vi "Measurement Main.vi"() -> ()   [LabVIEW 2017]
uses:
  Controls/saveDataOption.ctl
  TypeDefs/Trav-Command-TD.ctl
  Globals/measurementGlobal.vi
  <vilib>/Utility/file.llb/Read Delimited Spreadsheet (I64).vi
panel:
  in  "Boolean":bool
  in  "Trav Command":T1 items=["Set Reference", "Read Position", "Move", "StopMotors"]
  out "Traverse Position":i32[][](array[numeric])
  out "Block Index":i32
  in  "Setup":enum16{"Run Programme", "Show Setup"}(ring)
  in  "Data Acquisition":T2(ring)
  in  "Save Data Option":T3
  in  "Tap Control":enum32{"Plots", "Status and File"}(tab)
  out "Raw Signals":dbl[][](graph)
  in  "Folder Path":path
  out "Comments":string
  # "ON"
  # "OFF"
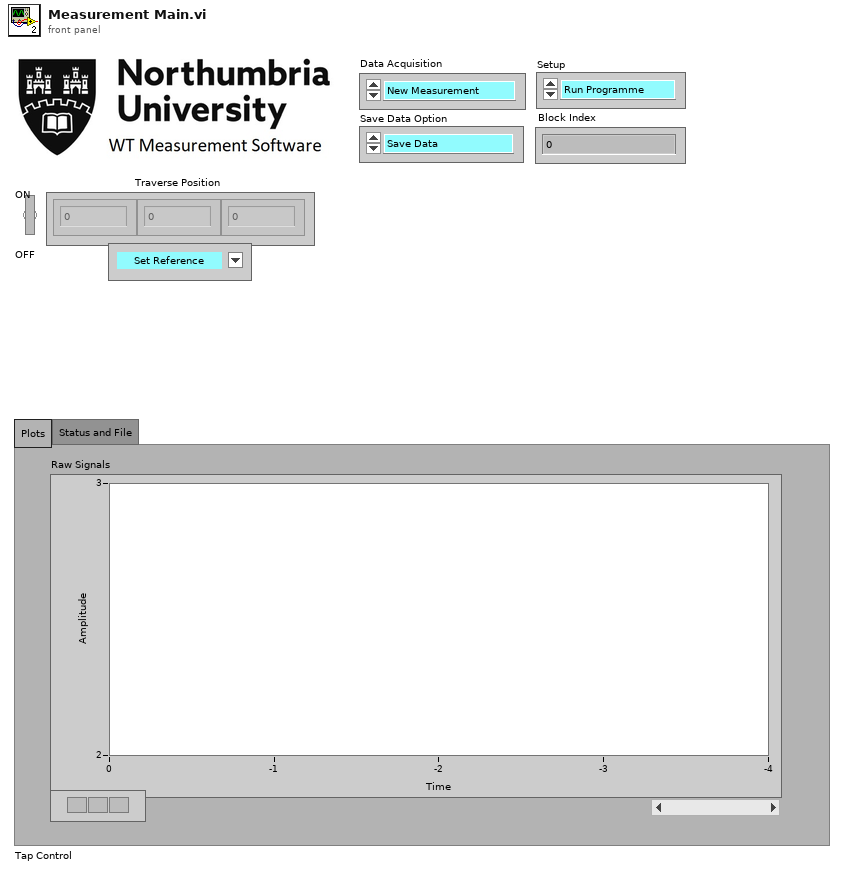
[diagram p1: front panel]
types:
  T1 = typedef "Trav-Command-TD.ctl" = u16
  T2 = enum16{"New Measurement", "Post-process Raw Data"}
  T3 = typedef "saveDataOption.ctl" = enum16{"Save Data", "Do Not Save Data"}
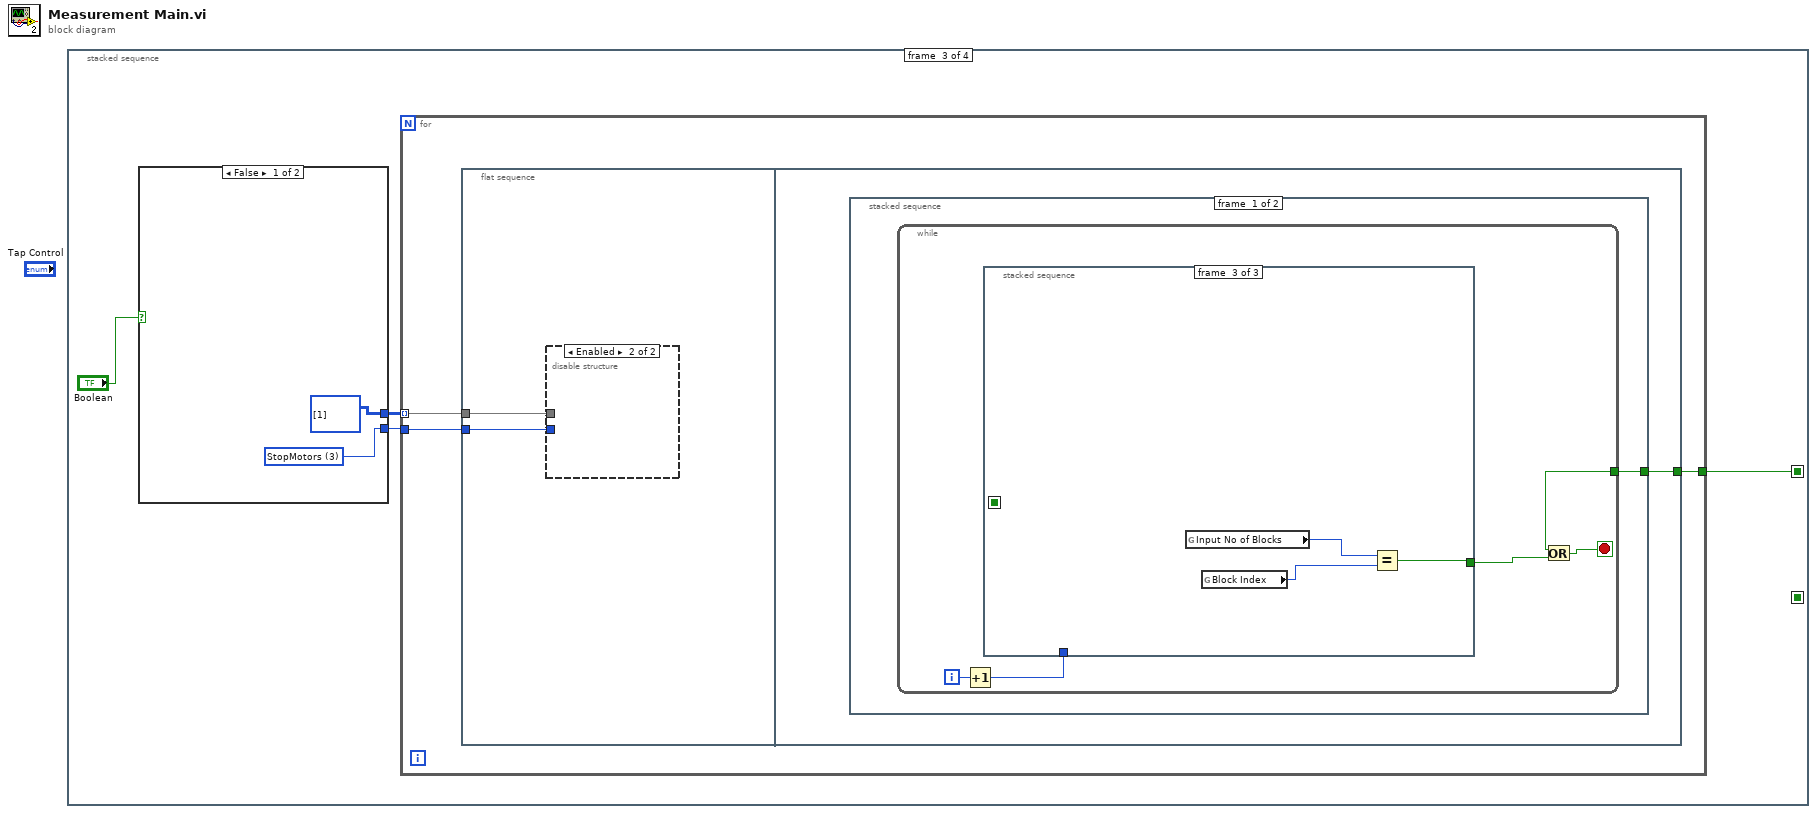
[diagram p0: block diagram]
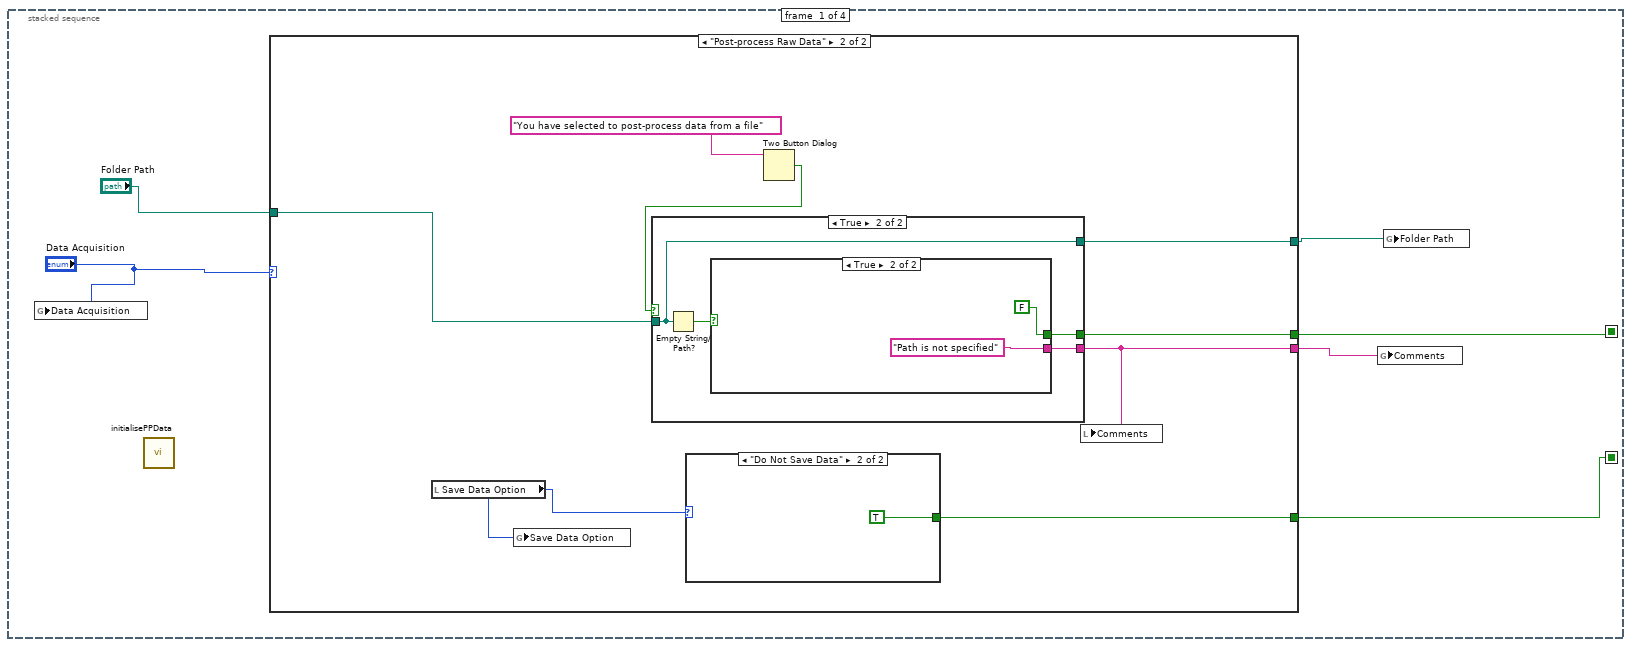
[diagram p2: hidden frame]
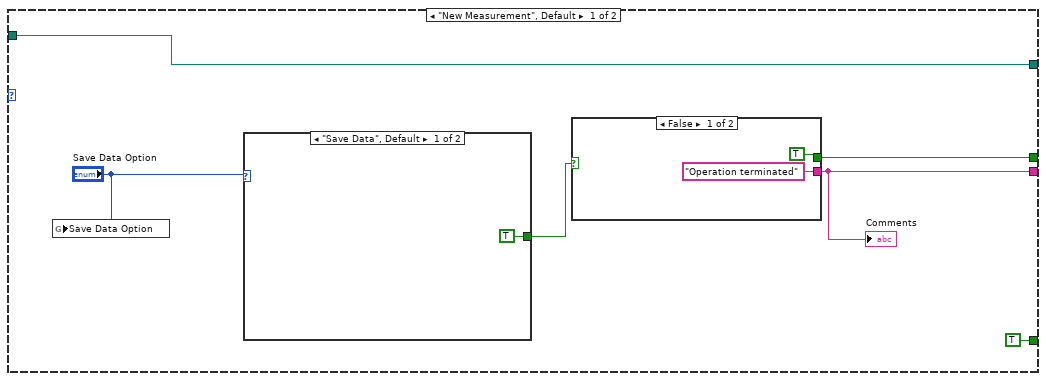
[diagram p3: hidden frame]
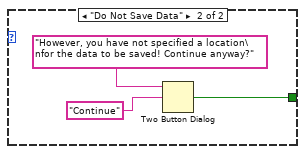
[diagram p4: hidden frame]
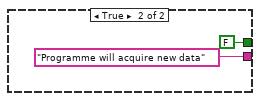
[diagram p5: hidden frame]
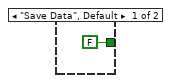
[diagram p6: hidden frame]
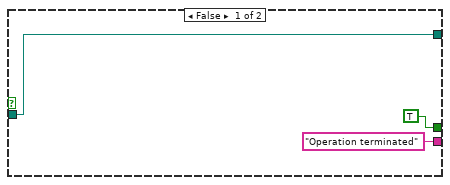
[diagram p7: hidden frame]
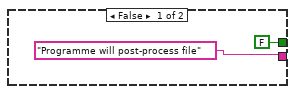
[diagram p8: hidden frame]
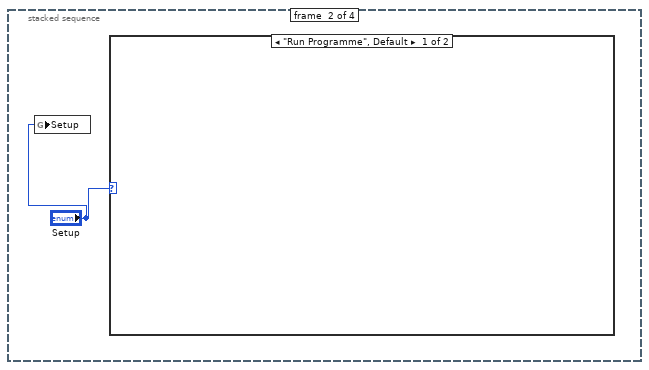
[diagram p9: hidden frame]
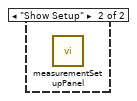
[diagram p10: hidden frame]
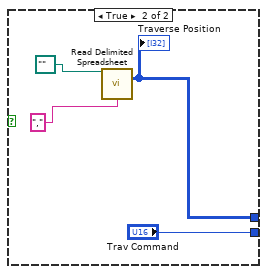
[diagram p11: hidden frame]
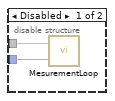
[diagram p12: hidden frame]
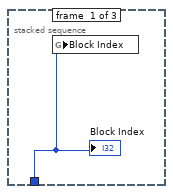
[diagram p13: hidden frame]
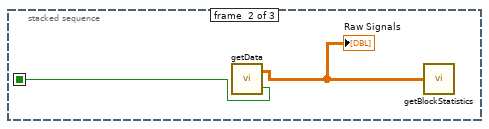
[diagram p14: hidden frame]
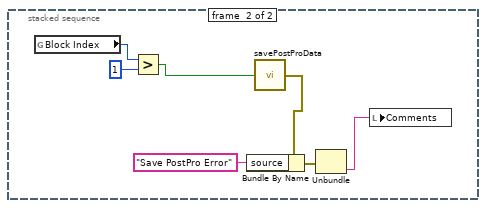
[diagram p15: hidden frame]
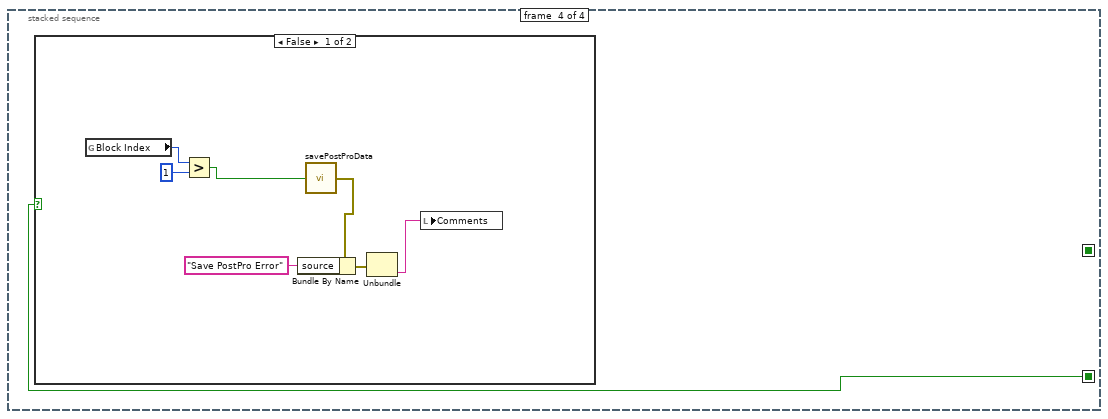
[diagram p16: hidden frame]
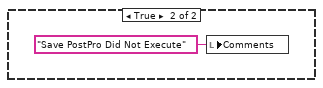
[diagram p17: hidden frame]
diagram:
  n1 = stacked-sequence {
    seq-local: [w4 _ _ _] -> [_ _ w46 _]
    seq-local: [w1 _ _ _] -> [_ _ _ w80]
    frame #0 {
      n2 = global write "measurementGlobal.vi" "Data Acquisition"("Data Acquisition") -> ()
      n3 = call "initialisePPData.vi"() -> ()  [unwired: 12 in]
      n4 = case shown="\"Post-process Raw Data\"" "Data Acquisition" {
        tunnel: [w10 w23] -> w6
        tunnel: [w12 w24] -> w4
        tunnel: "Folder Path" -> [w11 w26]
        tunnel: [w11 w25] -> w5
        tunnel: [TRUE w21] -> w1
        frame "New Measurement", Default {
          n5 = global write "measurementGlobal.vi" "Save Data Option"("Save Data Option") -> ()
          n6 = case shown="\"Save Data\", Default" "Save Data Option" {
            tunnel: [TRUE ("T button?") w15] -> w8
            frame "Save Data", Default {
            }
            frame "Do Not Save Data" {
              n7 = Two Button Dialog(message="However, you have not specified a location\nfor the data to be saved! Continue anyway?", 2:"Continue" ("T button name (\"OK\")")) -> (T button?=w15:bool)  [unwired: 1 in]
            }
          }
          n8 = case shown="False" w8 {
            tunnel: ["Operation terminated" ("Comments") "Programme will acquire new data" ("Comments")] -> w10
            tunnel: [TRUE FALSE] -> w12
            frame False {
            }
            frame True {
            }
          }
          "Comments" <- w10
        }
        frame "Post-process Raw Data" {
          n9 = local read "Save Data Option"() -> (w22:T3)
          n10 = global write "measurementGlobal.vi" "Save Data Option"(w22) -> ()
          n11 = case shown="\"Do Not Save Data\"" w22 {
            tunnel: [FALSE TRUE] -> w21
            frame "Save Data", Default {
            }
            frame "Do Not Save Data" {
            }
          }
          n12 = Two Button Dialog(message="You have selected to post-process data from a file") -> (T button?=w27:bool)  [unwired: 2 in]
          n13 = case shown="True" w27 {
            tunnel: w26 -> [w33 w35]
            tunnel: ["Operation terminated" w36] -> w23
            tunnel: [w33 w35] -> w25
            tunnel: [TRUE w34] -> w24
            frame False {
            }
            frame True {
              n14 = Empty String/Path?(string/path=w35) -> (empty?=w37:bool)
              n15 = case shown="True" w37 {
                tunnel: ["Programme will post-process file" "Path is not specified"] -> w36
                tunnel: [FALSE FALSE] -> w34
                frame False {
                }
                frame True {
                }
              }
            }
          }
          n16 = local write "Comments"(w23) -> ()
        }
      }
      n17 = global write "measurementGlobal.vi" "Comments"(w6) -> ()
      n18 = global write "measurementGlobal.vi" "Folder Path"(w5) -> ()
    }
    frame #1 {
      n19 = global write "measurementGlobal.vi" "Setup"("Setup") -> ()
      n20 = case shown="\"Run Programme\", Default" "Setup" {
        frame "Run Programme", Default {
        }
        frame "Show Setup" {
          n21 = call "measurementSetupPanel.vi"() -> ()  [unwired: 12 in]
        }
      }
    }
    frame #2 {
      n22 = case shown="False" "Boolean" {
        tunnel: [w48 "Trav Command"] -> w45
        tunnel: [i64[][] [[1]] ("all rows") w49] -> w44
        frame False {
          w48 = T1 3 items=["Set Reference", "Read Position", "Move", "StopMotors"] ("Trav Command")
        }
        frame True {
          n23 = call-poly <vilib>:"Read Delimited Spreadsheet.vi"("file path (dialog if empty)"=path "", "delimiter (\\t)"="," ("delimiter (\\t)")) -> ("all rows"=w49:i64[][])  [unwired: 8 in, 5 out]
          "Traverse Position" <- w49
        }
      }
      n24 = for {
        tunnel: w46 -> [w55]
        tunnel: w44 -> [w54] mode=indexing
        tunnel: w45 -> [w53]
        n25 = flat-sequence {
          tunnel: w54 -> [w57]
          tunnel: w53 -> [w56]
          tunnel: w55 -> [w60]
          frame #0 {
            n26 = disable-structure shown="Enabled" {
              disable-tunnel: w57 -> [w59 _]
              disable-tunnel: w56 -> [w58 _]
              frame Disabled {
                n27 = call "MesurementLoop.vi"("Trav Command"=w58, "All Rows"=w59) -> ()  [unwired: 1 in]
              }
              frame Enabled {
              }
            }
          }
          frame #1 {
            n28 = stacked-sequence {
              tunnel: w60 -> [w61 _]
              frame #0 {
                n29 = while {
                  tunnel: w61 -> [w64]
                  i -> [w66]
                  stop <- w62 stop-if-true
                  n30 = Increment(x=w66) -> (x+1=w65:i32)
                  n31 = stacked-sequence {
                    seq-local: [_ w69 _] -> [_ _ _]
                    tunnel: w65 -> [w67 _ _]
                    tunnel: [_ _ w70] -> w63
                    frame #0 {
                      n32 = global write "measurementGlobal.vi" "Block Index"(w67) -> ()
                      "Block Index" <- w67
                    }
                    frame #1 {
                      n33 = call "getData.vi"() -> ("Analogue Data (volts)"=w68:dbl[][], "Error Status"=w69:bool)  [unwired: 1 in]
                      "Raw Signals" <- w68
                      n34 = call "getBlockStatistics.vi"("Analogue Data (volts)"=w68) -> ()  [unwired: 1 out]
                    }
                    frame #2 {
                      n35 = global read "measurementGlobal.vi" "Input No of Blocks"() -> (w72:i32)
                      n36 = global read "measurementGlobal.vi" "Block Index"() -> (w71:i32)
                      n37 = Equal?(x=w72, y=w71) -> (x = y?=w70:bool)
                    }
                  }
                  n38 = Or(x=w64, y=w63) -> (x .or. y?=w62:bool)
                }
              }
              frame #1 {
                n39 = global read "measurementGlobal.vi" "Block Index"() -> (w79:i32)
                n40 = Greater?(x=w79, y=1) -> (0:w77:bool)
                n41 = call "savePostProData.vi"("append to file?"=w77) -> ("error out"=w75:errorcluster)  [unwired: 2 in]
                n42 = Bundle By Name(cluster=w75, "source"="Save PostPro Error") -> (w74:errorcluster)
                n43 = Unbundle(w74) -> ("source"=w73:string)  [unwired: 2 out]
                n44 = local write "Comments"(w73) -> ()
              }
            }
          }
        }
      }
    }
    frame #3 {
      n45 = case shown="False" w80 {
        frame False {
          n46 = global read "measurementGlobal.vi" "Block Index"() -> (w87:i32)
          n47 = Greater?(x=w87, y=1) -> (0:w85:bool)
          n48 = call "savePostProData.vi"("append to file?"=w85) -> ("error out"=w83:errorcluster)  [unwired: 2 in]
          n49 = Bundle By Name(cluster=w83, "source"="Save PostPro Error") -> (w82:errorcluster)
          n50 = Unbundle(w82) -> ("source"=w81:string)  [unwired: 2 out]
          n51 = local write "Comments"(w81) -> ()
        }
        frame True {
          n52 = local write "Comments"("Save PostPro Did Not Execute" ("Comments")) -> ()
        }
      }
    }
  }
